vi "Write.vi"(8 "error in (no error)":errorcluster, 10 "PV":refnum<class "PV.lvclass">, 11 "PVConnection in":refnum<class "PVConnection.lvclass">) -> (0 "error out":errorcluster, 3 "PVConnection out":refnum<class "PVConnection.lvclass">)   [LabVIEW 2012, in "CS++ProcessVariables.lvlib" / "PVConnection.lvclass"]
doc: "Publish a process varibale."
uses:
  PVConnection.lvclass
  ProcessVariable/PV.lvclass
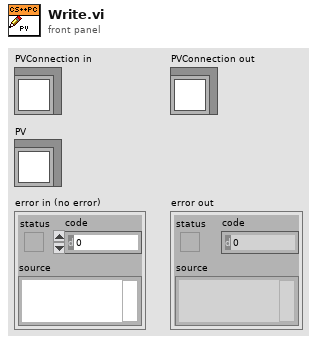
[diagram p1: front panel]
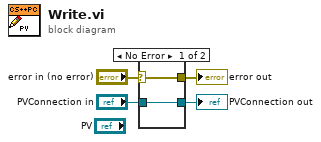
[diagram p0: block diagram]
diagram:
  n1 = case shown="No Error" "error in (no error)" {
    selector: "error in (no error)" -> [w5 w8]
    tunnel: [w5 w8] -> w3
    tunnel: [w6 w7] -> w1
    tunnel: "PVConnection in" -> [w6 w7]
    frame No Error {
    }
    frame Error {
    }
  }
  "error out" <- w3
  "PVConnection out" <- w1
